vi "send new command.vi"(10 "number":dbl, 11 "string":string) -> (3 "String":string)   [LabVIEW 2011, in "MoveDataFile.lvclass"]
uses:
  MoveDataFile.lvclass
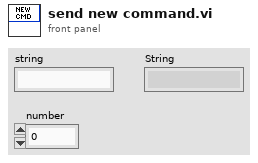
[diagram p1: front panel]
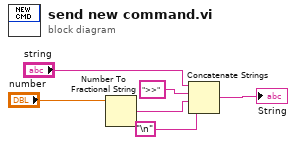
[diagram p0: block diagram]
diagram:
  n1 = Number To Fractional String(number="number") -> (F-format string=w3:string)  [unwired: 3 in]
  n2 = Concatenate Strings("string", ">>" ("string"), w3, "\n") -> (→"String":string)
